vi "Save_2D_Array.vi"(9 "Array":dbl[][](array[numeric]), 11 "Save":bool) -> ()   [LabVIEW 2013]
uses:
  <vilib>/Utility/file.llb/Write To Spreadsheet File (DBL).vi
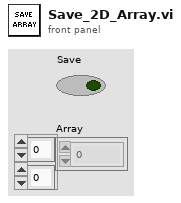
[diagram p1: front panel]
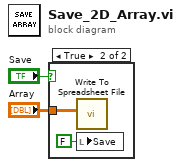
[diagram p0: block diagram]
diagram:
  n1 = case shown="True" "Save" {
    tunnel: "Array" -> [_ w3]
    frame False {
    }
    frame True {
      n2 = call-poly <vilib>:"Write To Spreadsheet File.vi"("2D data"=w3) -> ()  [unwired: 7 in, 1 out]
      n3 = local write "Save"(FALSE) -> ()
    }
  }
